vi "StartTestSuite_AfterEndTest_ReturnsNoError.vi"() -> (0 "error out":errorcluster)   [LabVIEW 2017, in "ResultTreeListener.Tests.lvlib"]
uses:
  ResultTreeListener.Tests.lvlib
  Support/FakeTestCase/FakeTestCase.lvclass
  C:/Users/de200256/Code/logmanoriginal/lvunit/Test/Test.lvclass
  Support/FakeTestSuite/FakeTestSuite.lvclass
  C:/Users/de200256/Code/logmanoriginal/lvunit/TestSuite/TestSuite.lvclass
  ResultTreeListener/ResultTreeListener.lvclass
  ResultTree/ResultTree.lvclass
  Assertion/Assertion.lvlib
panel:
  in  "Tree":string(tree)
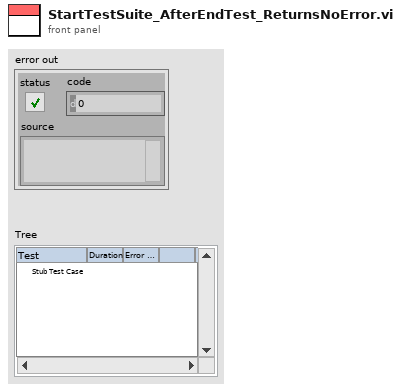
[diagram p1: front panel]
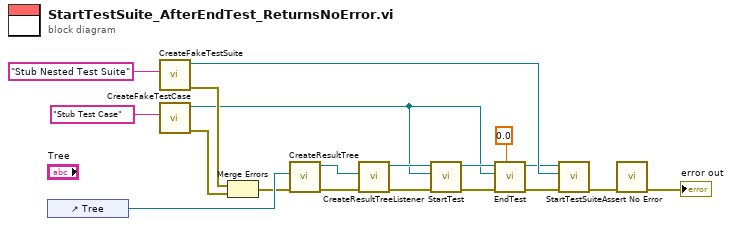
[diagram p0: block diagram]
diagram:
  n1 = control-ref of="Tree"() -> (w13:refnum<vi>)
  n2 = call "CreateFakeTestSuite.vi"("Name"="Stub Nested Test Suite") -> ("error out"=w8:errorcluster, "FakeTestSuite out"=w10:refnum<class "FakeTestSuite.lvclass">)  [unwired: 9 in]
  n3 = call "CreateFakeTestCase.vi"("Name"="Stub Test Case") -> ("error out"=w7:errorcluster, "FakeTestCase out"=w2:refnum<class "FakeTestCase.lvclass">)  [unwired: 9 in]
  n4 = Merge Errors(w8, w7) -> (w9:errorcluster)
  n5 = call "CreateResultTree.vi"("error in (no error)"=w9, "Tree Refnum"=w13) -> ("error out"=w19:errorcluster, "ResultTree out"=w18:refnum<class "ResultTree.lvclass">)  [unwired: 8 in]
  n6 = call "CreateResultTreeListener.vi"("error in (no error)"=w19, "ResultTree"=w18) -> ("error out"=w17:errorcluster, "ResultTreeListener out"=w15:refnum<class "ResultTreeListener.lvclass">)  [unwired: 8 in]
  n7 = call-dynamic "StartTest.vi"("error in (no error)"=w17, "Test"=w2, "ResultTreeListener in"=w15) -> ("error out"=w11:errorcluster, "ResultTreeListener out"=w4:refnum<class "ResultTreeListener.lvclass">)  [unwired: 7 in]
  n8 = call-dynamic "EndTest.vi"("Time"=0.0, "error in (no error)"=w11, "Test"=w2, "ResultTreeListener in"=w4) -> ("error out"=w5:errorcluster, "ResultTreeListener out"=w3:refnum<class "ResultTreeListener.lvclass">)  [unwired: 6 in]
  n9 = call-dynamic "StartTestSuite.vi"("error in (no error)"=w5, "TestSuite"=w10, "ResultTreeListener in"=w3) -> ("error out"=w6:errorcluster)  [unwired: 7 in, 1 out]
  n10 = call "Assert No Error.vi"("error in (no error)"=w6) -> ("error out"=→"error out":errorcluster)  [unwired: 10 in]
